vi "Set Config.vi"(8 "error in (no error)":errorcluster, 11 "Configur":T1) -> (0 "error out":errorcluster)   [LabVIEW 2025, in "Full User Interface.lvlib"]
uses:
  Full User Interface.lvlib
  <vilib>/Test Bench Framework/Test Executive.lvlibp/TestEngine/TestEngine/TestEngine/Typedefs/TestEngine Cofiguration.ctl
  <vilib>/Test Bench Framework/Test Executive.lvlibp/TestEngine/TestEngine/TestEngine/Typedefs/Local Report Configuration.ctl
  <vilib>/Test Bench Framework/Test Executive.lvlibp/TestEngine/TestEngine/TestEngine/Report Format.ctl
  <vilib>/Test Bench Framework/Test Executive.lvlibp/TestEngine/TestEngine/TestEngine/Typedefs/Database Configuration.ctl
  <vilib>/Utility/config.llb/NI_LVConfig.lvlib
  <userlib>/_OpenG.lib/variantconfig/variantconfig.llb/openg_variant_configuration_file.lvlib
  <vilib>/Test Bench Framework/Test Executive.lvlibp/TestEngine/TestEngine/TestEngine/Test Engine.lvclass
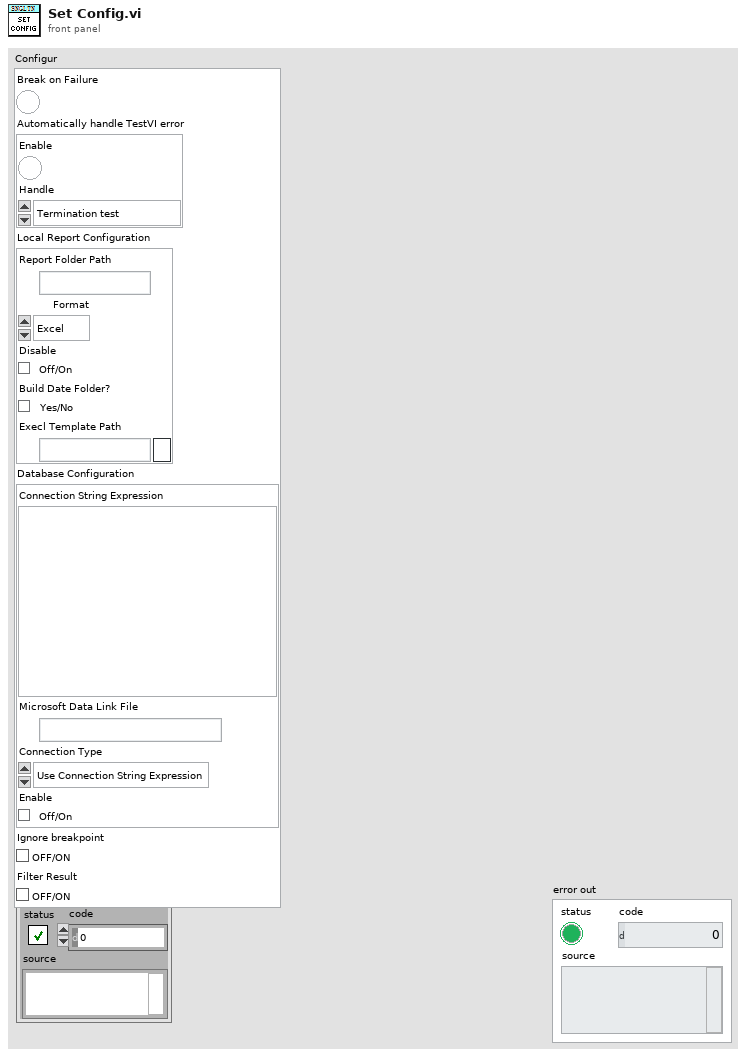
[diagram p1: front panel]
types:
  T1 = typedef "Test Executive.lvlibp/Test Engine.lvlib/Test Engine.lvclass/TestEngine Cofiguration.ctl" = cluster{"Break on Failure":bool, "Automatically handle TestVI error":cluster{"Enable":bool, "Handle":enum16{"Termination test", "Ignore error"}}, "Local Report Configuration":T2, "Database Configuration":T4, "Ignore breakpoint":bool, "Filter Result":bool}
  T2 = typedef "Test Executive.lvlibp/Test Engine.lvlib/Test Engine.lvclass/Local Report Configuration.ctl" = cluster{"Report Folder Path":path, "Format":T3, "Disable":bool, "Build Date Folder?":bool, "Execl Template Path":path}
  T3 = typedef "Test Executive.lvlibp/Test Engine.lvlib/Test Engine.lvclass/Report Format.ctl" = enum16{"Excel", "CSV(Tab)", "CSV(,)", "CSV(;)", "TEXT", "HTML"}
  T4 = typedef "Test Executive.lvlibp/Test Engine.lvlib/Test Engine.lvclass/Database Configuration.ctl" = cluster{"Connection String Expression":string, "Microsoft Data Link File":path, "Connection Type":enum16{"Use Connection String Expression", "Use Microsoft Data Link File"}, "Enable":bool}
  T5 = typedef "NI_LVConfig.lvlib/Config Data RefNum.ctl" = refnum<k1>
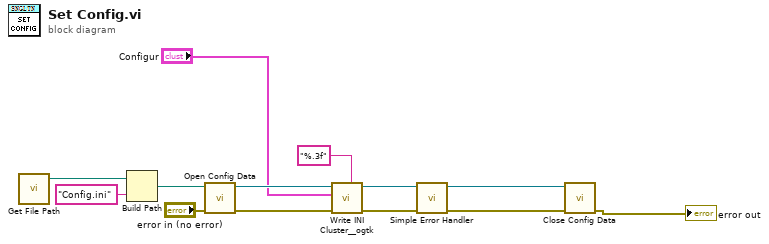
[diagram p0: block diagram]
diagram:
  n1 = call "Get File Path.vi"() -> ("Application Directory"=w10:path)  [unwired: 11 in]
  n2 = Build Path(base path=w10, name or relative path="Config.ini") -> (appended path=w8:path)
  n3 = call <vilib>:"Open Config Data.vi"("error in (no error)"="error in (no error)", "configuration file path"=w8) -> ("error out"=w11:errorcluster, "refnum"=w12:T5)  [unwired: 7 in, 1 out]
  n4 = call <userlib>:"Write INI Cluster__ogtk.vi"("float number format (optional)"="%.3f", "error in (no error)"=w11, "INI Fomatted Cluster"="Configur", "refnum"=w12) -> ("error out"=w6:errorcluster, "dup refnum"=w7:T5)  [unwired: 6 in]
  n5 = call <vilib>:"Simple Error Handler.vi"("error in (no error)"=w6) -> ("error out"=w1:errorcluster)  [unwired: 4 in, 4 out]
  n6 = call <vilib>:"Close Config Data.vi"("error in (no error)"=w1, "refnum"=w7) -> ("error out"=→"error out":errorcluster)  [unwired: 8 in, 1 out]
